vi "AnalyzeSpectrum.vi"(8 "error in (no error)":errorcluster, 9 "data":T1, 11 "config":T5[](array[typedef])) -> (0 "error out":errorcluster, 1 "data out":T1)   [LabVIEW 2017, in "EmsaAnalysis.lvlib"]
uses:
  <vilib>/addons/InsightCM/Devices/Shared/Emsa/EmsaAnalysis/EmsaAnalysis.lvlib
  <vilib>/addons/InsightCM/Devices/Shared/Emsa/EmsaAnalysis/controls/datagroupMetrics.ctl
  <vilib>/addons/InsightCM/Devices/Shared/Emsa/EmsaAnalysis/controls/channelMetrics.ctl
  <vilib>/addons/InsightCM/Devices/Shared/Emsa/EmsaAnalysis/controls/metric.ctl
  <vilib>/addons/InsightCM/MessageBus/Base/controls/MetricDefinitionInstance.ctl
  <vilib>/addons/InsightCM/MessageBus/Base/controls/KeyValuePair.ctl
  <vilib>/addons/InsightCM/Devices/Shared/Emsa/EmsaAnalysis/controls/sweepInfo.ctl
  <vilib>/addons/InsightCM/Devices/Shared/Common/DataFlow/controls/Data.ctl
  <vilib>/addons/InsightCM/Utilities/DataAccessors/controls/wfmSGL_DVR.ctl
  <vilib>/addons/PointValueMap/controls/PointMap.ctl
  <vilib>/addons/InsightCM/Devices/Shared/Common/DataFlow/controls/Type.ctl
  <vilib>/addons/PointValueMap/subVIs/Point_Write_double.vi
  <vilib>/addons/PointValueMap/PointValueMap.lvlib
  <vilib>/addons/InsightCM/Utilities/PropertyHelpers/PropertyHelpers.lvlib
  <vilib>/addons/InsightCM/Devices/Shared/Emsa/EmsaAcquisition/EmsaAcquisition.lvlib
  <vilib>/addons/InsightCM/Devices/Shared/Common/DataFlow/DataFlow.lvlib
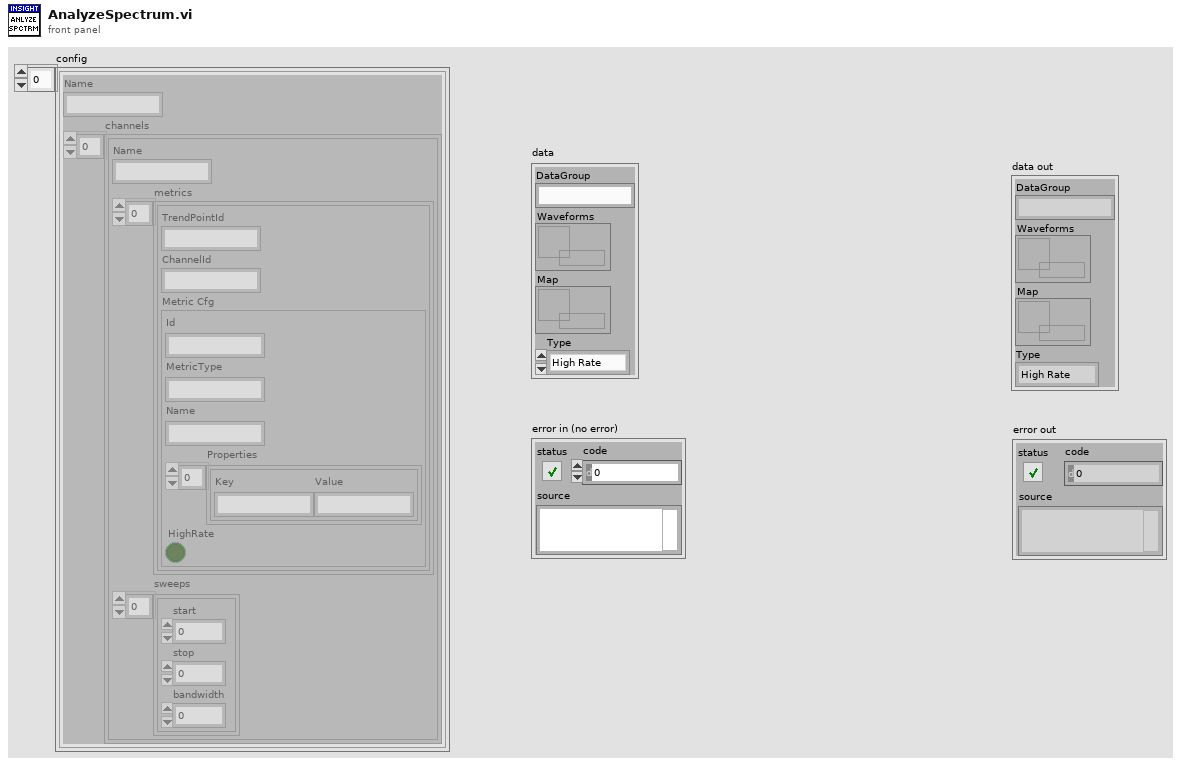
[diagram p1: front panel]
types:
  T1 = typedef "DataFlow.lvlib/Data.ctl" = cluster{"DataGroup":string, "Waveforms":T2, "Map":T3, "Type":T4}
  T2 = typedef "wfmSGL_DVR.ctl" = refnum<data-value>
  T3 = typedef "PointValueMap.lvlib/PointMap.ctl" = refnum<data-value>
  T4 = typedef "DataFlow.lvlib/Type.ctl" = enum16{"High Rate", "Low Rate", "Burst Mode"}
  T5 = typedef "EmsaAnalysis.lvlib/datagroupMetrics.ctl" = cluster{"Name":string, "channels":T6[]}
  T6 = typedef "EmsaAnalysis.lvlib/channelMetrics.ctl" = cluster{"Name":string, "metrics":T7[], "sweeps":T10[]}
  T7 = typedef "EmsaAnalysis.lvlib/metric.ctl" = cluster{"TrendPointId":string, "ChannelId":string, "Metric Cfg":T8}
  T8 = typedef "MetricDefinitionInstance.ctl" = cluster{"Id":string, "MetricType":string, "Name":string, "Properties":T9[], "HighRate":bool}
  T9 = typedef "KeyValuePair.ctl" = cluster{"Key":string, "Value":string}
  T10 = typedef "EmsaAnalysis.lvlib/sweepInfo.ctl" = cluster{"start":dbl, "stop":dbl, "bandwidth":dbl}
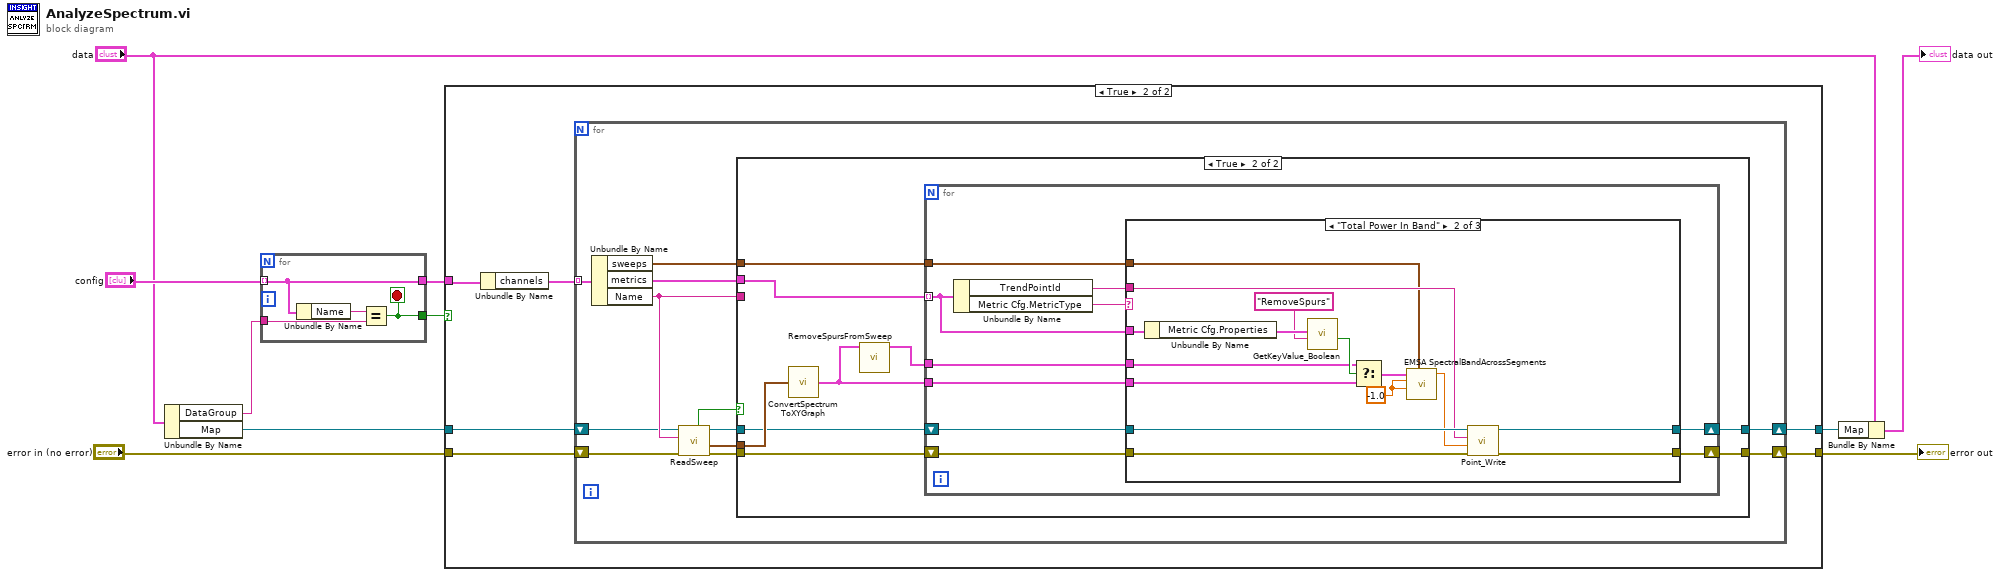
[diagram p0: block diagram]
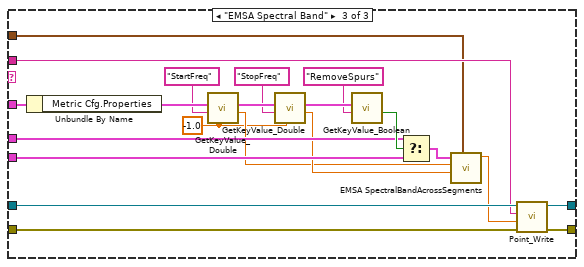
[diagram p5: hidden frame]
diagram:
  n1 = Unbundle By Name("data") -> ("DataGroup"=w9:string, "Map"=w3:T3)
  n2 = for {
    tunnel: "config" -> [w12] mode=indexing
    tunnel: w9 -> [w13]
    tunnel: [w12] -> w8
    tunnel: [w11] -> w4
    stop <- w11 stop-if-true
    n3 = Unbundle By Name(w12) -> ("Name"=w14:string)
    n4 = Equal?(x=w14, y=w13) -> (x = y?=w11:bool)
  }
  n5 = case shown="True" w4 {
    tunnel: w8 -> [_ w22]
    tunnel: w3 -> [w16 w20]
    tunnel: [w16 w17] -> w6
    tunnel: "error in (no error)" -> [w15 w19]
    tunnel: [w15 w18] -> w1
    frame False {
      # "datagroup not found"
    }
    frame True {
      n6 = Unbundle By Name(w22) -> ("channels"=w21:T6[])
      n7 = for {
        tunnel: w21 -> [w34] mode=indexing
        shift-right: [w31] -> w18
        shift-left: w19 -> [w28]
        shift-right: [w23] -> w17
        shift-left: w20 -> [w29]
        n8 = Unbundle By Name(w34) -> ("sweeps"=w32:T10[], "metrics"=w33:T7[], "Name"=w30:string)
        n9 = call <vilib>:"ReadSweep.vi"("error in (no error)"=w28, "channel"=w30, "map"=w29) -> ("error out"=w27:errorcluster, "sweep"=w26:cluster{"frequency":dbl, "amplitude":dbl}[], "map out"=w24:T3, "valid"=w25:bool)  [unwired: 3 in, 2 out]
        n10 = case shown="True" w25 {
          tunnel: w33 -> [_ w45]
          tunnel: [w35 w37] -> w23
          tunnel: w32 -> [_ w42]
          tunnel: w30 -> [_ _]
          tunnel: w27 -> [w36 w39]
          tunnel: [w36 w41] -> w31
          tunnel: w26 -> [_ w40]
          tunnel: w24 -> [w35 w38]
          frame False {
          }
          frame True {
            n11 = call <vilib>:"ConvertSpectrumToXYGraph.vi"("spectrum"=w40) -> ("xy graph"=w43:cluster{"frequency":dbl[], "amplitude":dbl[]})  [unwired: 4 in]
            n12 = call <vilib>:"RemoveSpursFromSweep.vi"("sweep"=w43) -> ("sweep"=w44:cluster{"frequency":dbl[], "amplitude":dbl[]})  [unwired: 10 in]
            n13 = for {
              tunnel: w45 -> [w54] mode=indexing
              tunnel: w42 -> [w51]
              tunnel: w44 -> [w50]
              tunnel: w43 -> [w49]
              shift-right: [w47] -> w41
              shift-left: w39 -> [w48]
              shift-right: [w46] -> w37
              shift-left: w38 -> [w53]
              n14 = Unbundle By Name(w54) -> ("TrendPointId"=w52:string, "Metric Cfg.MetricType"=w55:string)
              n15 = case shown="\"Total Power In Band\"" w55 {
                tunnel: w54 -> [_ w69 w90]
                tunnel: w53 -> [w57 w72 w93]
                tunnel: w52 -> [_ w71 w92]
                tunnel: [w57 w70 w91] -> w46
                tunnel: w51 -> [_ w61 w79]
                tunnel: w50 -> [_ w65 w82]
                tunnel: w49 -> [_ w64 w81]
                tunnel: w48 -> [w56 w59 w74]
                tunnel: [w56 w58 w73] -> w47
                frame "", Default {
                }
                frame "Total Power In Band" {
                  w60 = -1.0 ("start frequency")
                  n16 = Unbundle By Name(w69) -> ("Metric Cfg.Properties"=w68:T9[])
                  n17 = call <vilib>:"GetKeyValue_Boolean.vi"("key"="RemoveSpurs", "key value pairs"=w68) -> ("value"=w66:bool)  [unwired: 7 in, 2 out]
                  n18 = Select(t=w65, s=w66, f=w64) -> (s? t:f=w62:cluster{"frequency":dbl[], "amplitude":dbl[]})
                  n19 = call <vilib>:"EMSA SpectralBandAcrossSegments.vi"("sweeps"=w61, "stop frequency"=w60, "start frequency"=w60, "sweep in"=w62) -> ("power in band"=w63:dbl)  [unwired: 5 in, 2 out]
                  n20 = call-poly <vilib>:"Point_Write.vi"("Error In"=w59, "Value"=w63, "Tag"=w71, "Map"=w72) -> ("Error Out"=w58:errorcluster, "Map Out"=w70:T3)  [unwired: 6 in]
                }
                frame "EMSA Spectral Band" {
                  w76 = -1.0 ("default")
                  n21 = Unbundle By Name(w90) -> ("Metric Cfg.Properties"=w89:T9[])
                  n22 = call <vilib>:"GetKeyValue_Double.vi"("default"=w76, "key"="StartFreq", "key value pairs"=w89) -> ("value"=w77:dbl, "key value pairs out"=w87:T9[])  [unwired: 6 in, 1 out]
                  n23 = call <vilib>:"GetKeyValue_Double.vi"("default"=w76, "key"="StopFreq", "key value pairs"=w87) -> ("value"=w78:dbl, "key value pairs out"=w85:T9[])  [unwired: 6 in, 1 out]
                  n24 = call <vilib>:"GetKeyValue_Boolean.vi"("key"="RemoveSpurs", "key value pairs"=w85) -> ("value"=w83:bool)  [unwired: 7 in, 2 out]
                  n25 = Select(t=w82, s=w83, f=w81) -> (s? t:f=w80:cluster{"frequency":dbl[], "amplitude":dbl[]})
                  n26 = call <vilib>:"EMSA SpectralBandAcrossSegments.vi"("sweeps"=w79, "stop frequency"=w78, "start frequency"=w77, "sweep in"=w80) -> ("power in band"=w75:dbl)  [unwired: 5 in, 2 out]
                  n27 = call-poly <vilib>:"Point_Write.vi"("Error In"=w74, "Value"=w75, "Tag"=w92, "Map"=w93) -> ("Error Out"=w73:errorcluster, "Map Out"=w91:T3)  [unwired: 6 in]
                }
              }
            }
          }
        }
      }
    }
  }
  "error out" <- w1
  n28 = Bundle By Name(cluster="data", "Map"=w6) -> (→"data out":T1)
